vi "Clear Filters.vi"(8 "error in (no error)":errorcluster, 11 "Bus Monitor in":refnum<class "Bus Monitor.lvclass">) -> (0 "error out":errorcluster, 3 "Bus Monitor out":refnum<class "Bus Monitor.lvclass">)   [LabVIEW 2020, in "BCI-1553 API.lvlib" / "Bus Monitor.lvclass"]
doc: "Removes all the filters from this Bus Monitor."
uses:
  Bus Monitor.lvclass
  Bus Monitor.lvclass/Bus Monitor.ctl
  Dependencies/Registry/Registry.lvclass/Registry.ctl
  Dependencies/Registry/Registry.lvclass
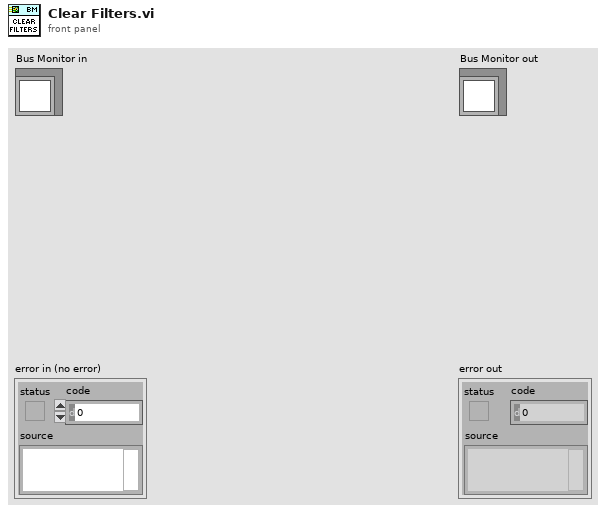
[diagram p1: front panel]
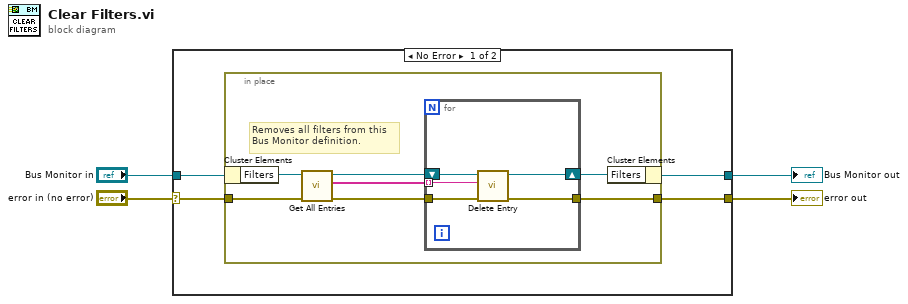
[diagram p0: block diagram]
diagram:
  n1 = case shown="No Error" "error in (no error)" {
    selector: "error in (no error)" -> [w5 w21]
    tunnel: [w6 w21] -> w1
    tunnel: [w7 w20] -> w2
    tunnel: "Bus Monitor in" -> [w8 w20]
    frame No Error {
      n2 = in-place {
        in-place-border: [w9] -> w6
        in-place-border: w5 -> [w14]
        # "Removes all filters from this\nBus Monitor definition."
        n3 = in-place-cluster #1(w8) -> ("Filters"=w12:refnum<class "Registry.lvclass">)
        n4 = call "Get All Entries.vi"("error in (no error)"=w14, "Registry in"=w12) -> ("error out"=w13:errorcluster, "Keys"=w11:string[])  [unwired: 7 in, 1 out]
        n5 = for {
          tunnel: w13 -> [w18]
          tunnel: w11 -> [w17] mode=indexing
          tunnel: [w15] -> w9
          shift-right: [w16] -> w10
          shift-left: w12 -> [w19]
          n6 = call "Delete Entry.vi"("error in (no error)"=w18, "Key"=w17, "Registry in"=w19) -> ("error out"=w15:errorcluster, "Registry out"=w16:refnum<class "Registry.lvclass">)  [unwired: 6 in, 1 out]
        }
        n7 = in-place-cluster #1("Filters"=w10) -> (w7:refnum<class "Bus Monitor.lvclass">)
      }
    }
    frame Error {
    }
  }
  "error out" <- w1
  "Bus Monitor out" <- w2
